vi "LV SciSDK CUSTOM PACKET STOP.vi"(8 "error in (no error)":errorcluster, 9 "CP Handle In":cluster{"CP Path":string, "CP Name":string}) -> (0 "error out":errorcluster, 1 "CP Handle Out":cluster{"CP Path":string, "CP Name":string}, 3 "NI Error Code":i32)   [LabVIEW 2021, in "SciSDK_Labview.lvlib"]
doc: "You need this VI to execute command to stop to generate custom packets"
uses:
  SciSDK_Labview.lvlib
panel:
  out "Board Handle Out":T1
  in  "Board Handle In":T1
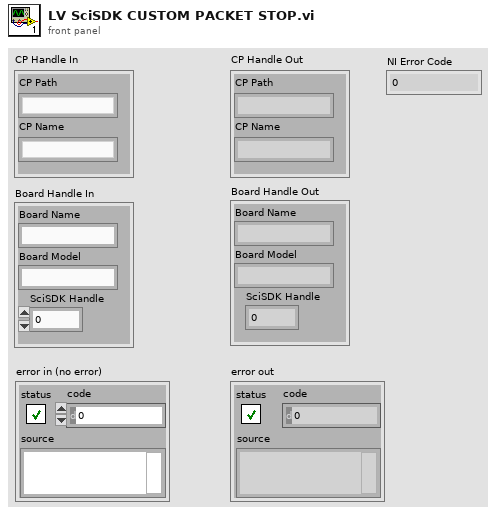
[diagram p1: front panel]
types:
  T1 = cluster{"Board Name":string, "Board Model":string, "SciSDK Handle":u64}
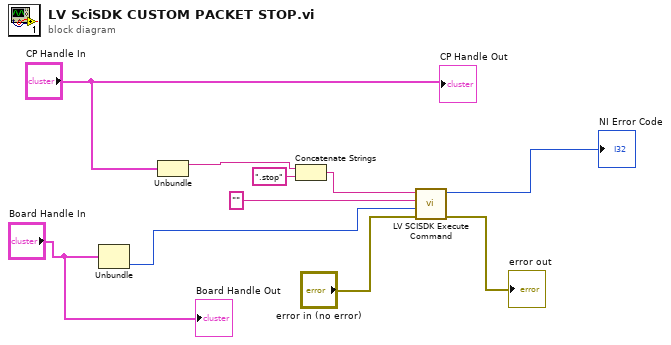
[diagram p0: block diagram]
diagram:
  n1 = Unbundle("Board Handle In") -> ("SciSDK Handle"=w2:u64)  [unwired: 2 out]
  n2 = Unbundle("CP Handle In") -> ("CP Path"=w3:string)  [unwired: 1 out]
  n3 = Concatenate Strings(w3, ".stop" ("string")) -> (w7:string)
  n4 = call "LV SCISDK Execute Command.vi"("error in (no error)"="error in (no error)", "handle"=w2, "value"="", "Path"=w7) -> ("error out"=→"error out":errorcluster, "function return"=→"NI Error Code":i32)  [unwired: 5 in, 1 out]
  "CP Handle Out" <- "CP Handle In"
  "Board Handle Out" <- "Board Handle In"
